vi "Counter - Finite Output.vi"() -> ()   [LabVIEW 2025]
doc: "This example demonstrates how to generate a finite number of digital pulses using a counter output.\n\nOn some hardware, this requires the use of a second counter to generate a gate signal. If necessary, DAQmx configures this second counter for you."
uses:
  <vilib>/Utility/error.llb/DialogType.ctl
  <vilib>/DAQmx/create/channels.llb/DAQmx Create Channel (CO-Pulse Generation-Time).vi
  <vilib>/DAQmx/configure/timing.llb/DAQmx Timing (Implicit).vi
  <vilib>/DAQmx/configure/trigger.llb/DAQmx Start Trigger (Digital Edge).vi
  <resource>/objmgr/daqmx.rc
panel:
  in  "Number of Pulses":i32=20
  in  "Low Time (ms)":dbl=0.02 format="%.6f"
  in  "High Time (ms)":dbl=0.02 format="%.6f"
  in  "Output Terminal":tag="/PXI1Slot8/PFI0"
  in  "Trigger Type":enum32{"No Trigger", "Digital Start"}(tab)
  in  "Retriggerable":bool
  in  "Edge":i32(ring)=10280 items=["Rising"=10280, "Falling"=10171]
  in  "Digital Trigger Source":tag
  in  "Stop":bool
  in  "Counter":tag="PXI1Slot8/ctr0"
  # "Channel Settings"
  # "Timing Settings"
  # "Trigger Settings"
  # "To configure and use a trigger you must have the necessary tab selected above."
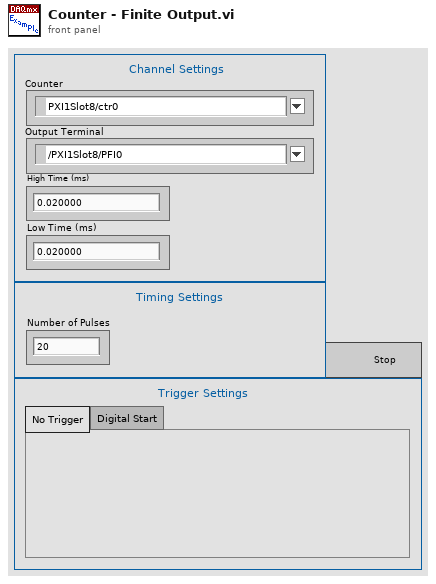
[diagram p1: front panel]
types:
  T1 = typedef "DialogType.ctl" = u16
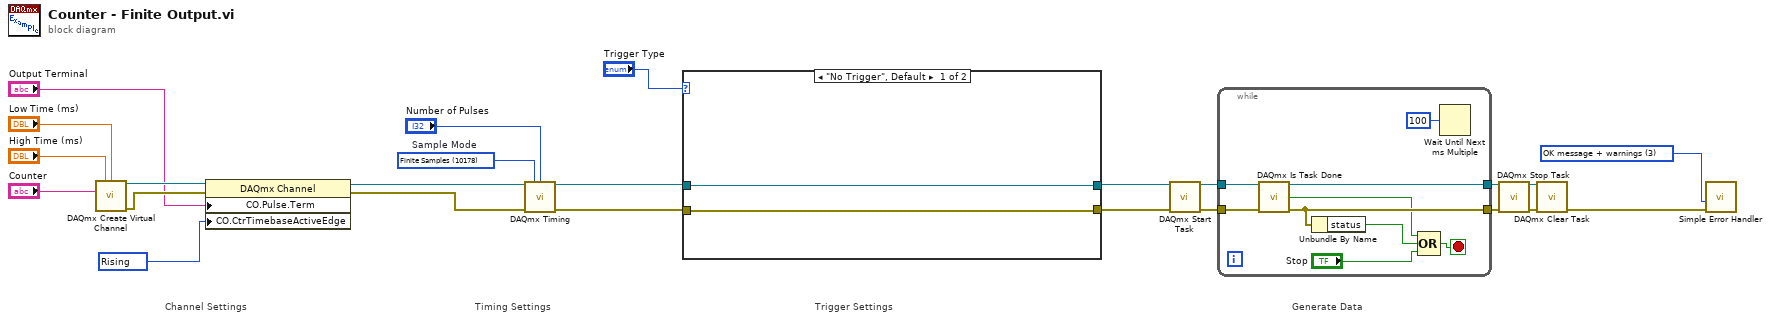
[diagram p0: block diagram]
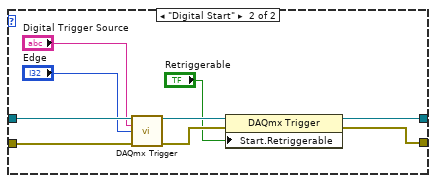
[diagram p2: hidden frame]
diagram:
  w1 = 10280 items=["Rising"=10280, "Falling"=10171] ("CO.CtrTimebaseActiveEdge")
  w2 = T1 3 items=["no dialog", "OK message", "continue or stop message", "OK message + warnings", "continue/stop + warnings"] ("type of dialog (OK msg:1)")
  w24 = 10178 items=["Finite Samples"=10178, "Continuous Samples"=10123, "Hardware Timed Single Point"=12522]  # Sample Mode
  # "Generate Data"
  # "Trigger Settings"
  # "Timing Settings"
  # "Channel Settings"
  n1 = call-poly <vilib>:"DAQmx Create Virtual Channel.vi"("high time"="High Time (ms)", "low time"="Low Time (ms)", "counter"="Counter") -> ("task out"=w14:refnum<k21>, "error out"=w13:errorcluster)  [unwired: 11 in]
  n2 = property class="DAQmx Channel"(reference=w14, error in=w13, "CO.Pulse.Term"="Output Terminal", "CO.CtrTimebaseActiveEdge"=w1) -> (reference out=w10:refnum<k21>, error out=w11:errorcluster)
  n3 = call-poly <vilib>:"DAQmx Timing.vi"("task/channels in"=w10, "sample mode"=w24, "samples per channel"="Number of Pulses", "error in"=w11) -> ("task out"=w18:refnum<k21>, "error out"=w17:errorcluster)  [unwired: 10 in]
  n4 = case shown="\"No Trigger\", Default" "Trigger Type" {
    tunnel: w18 -> [w26 w35]
    tunnel: w17 -> [w25 w34]
    tunnel: [w26 w31] -> w15
    tunnel: [w25 w30] -> w16
    frame "No Trigger", Default {
    }
    frame "Digital Start" {
      n5 = call-poly <vilib>:"DAQmx Trigger.vi"("task/channels in"=w35, "source"="Digital Trigger Source", "edge"="Edge", "error in"=w34) -> ("task out"=w28:refnum<k21>, "error out"=w29:errorcluster)  [unwired: 10 in]
      n6 = property class="DAQmx Trigger"(reference=w28, error in=w29, "Start.Retriggerable"="Retriggerable") -> (reference out=w31:refnum<k21>, error out=w30:errorcluster)
    }
  }
  n7 = call <vilib>:"DAQmx Start Task.vi"("task/channels in"=w15, "error in"=w16) -> ("task out"=w23:refnum<k21>, "error out"=w22:errorcluster)  [unwired: 12 in]
  n8 = while {
    tunnel: w23 -> [w44]
    tunnel: w22 -> [w43]
    tunnel: [w40] -> w3
    tunnel: [w41] -> w4
    stop <- w42 stop-if-true
    n9 = call <vilib>:"DAQmx Is Task Done.vi"("task/channels in"=w44, "error in"=w43) -> ("task out"=w41:refnum<k21>, "task done?"=w36:bool, "error out"=w40:errorcluster)  [unwired: 11 in]
    n10 = Unbundle By Name(w40) -> ("status"=w39:bool)
    n11 = Compound Arithmetic op=OR(w36, w39, "Stop") -> (w42:bool)
    n12 = Wait Until Next ms Multiple(millisecond multiple=u32 100) -> ()  [unwired: 1 out]
  }
  n13 = call <vilib>:"DAQmx Stop Task.vi"("task/channels in"=w4, "error in"=w3) -> ("task out"=w6:refnum<k21>, "error out"=w5:errorcluster)  [unwired: 12 in]
  n14 = call <vilib>:"DAQmx Clear Task.vi"("task in"=w6, "error in"=w5) -> ("error out"=w21:errorcluster)  [unwired: 13 in]
  n15 = call <vilib>:"Simple Error Handler.vi"("type of dialog (OK msg:1)"=w2, "error in (no error)"=w21) -> ()  [unwired: 3 in, 5 out]
